vi "MAINrx.vi"() -> ()   [LabVIEW 2017]
uses:
  <instrlib>/niUSRP/niUSRP Write Tx Data (CDB).vi
panel:
  in  "SYNCHRO":i8[](array[numeric])=[0, 1, 1, 0, 1, 0, 0, 0, 0, 0, 0, 0, 1, 0, 0, 0, 0, 0, 1, 1]
  in  "simbol per write":i32=120
  out "Numeric":i32=3141
  out "cicli 2":dbl=18.0
  out "cicli":dbl=19.0
  in  "Silent symbol":i32=70
  in  "trama length":i32=20000
  out "original data  array":u16[](array[numeric])
  out "size(s)":i32=375000
  in  "Color":bool=TRUE
  out "Image out":T1(plugin-control)
  in  "Enabled Channel":string(combo)="0"
  in  "Device Name":refnum<k15>="192.168.10.2"
  in  "Active Antenna":string="TX1"
  in  "Gain":dbl=100.0 format="%#_6f"
  in  "Carrier Frequency":dbl format="%#_6p"
  in  "IQ Rate":dbl=2000000.0 format="%#_6p"
  in  "File Path":path=path "C:/Users/33769/Desktop/San-Giovanni-in-Fiore-Cosenza.jpg"
  in  "M":i32=16
  in  "pulse duration":i32=5
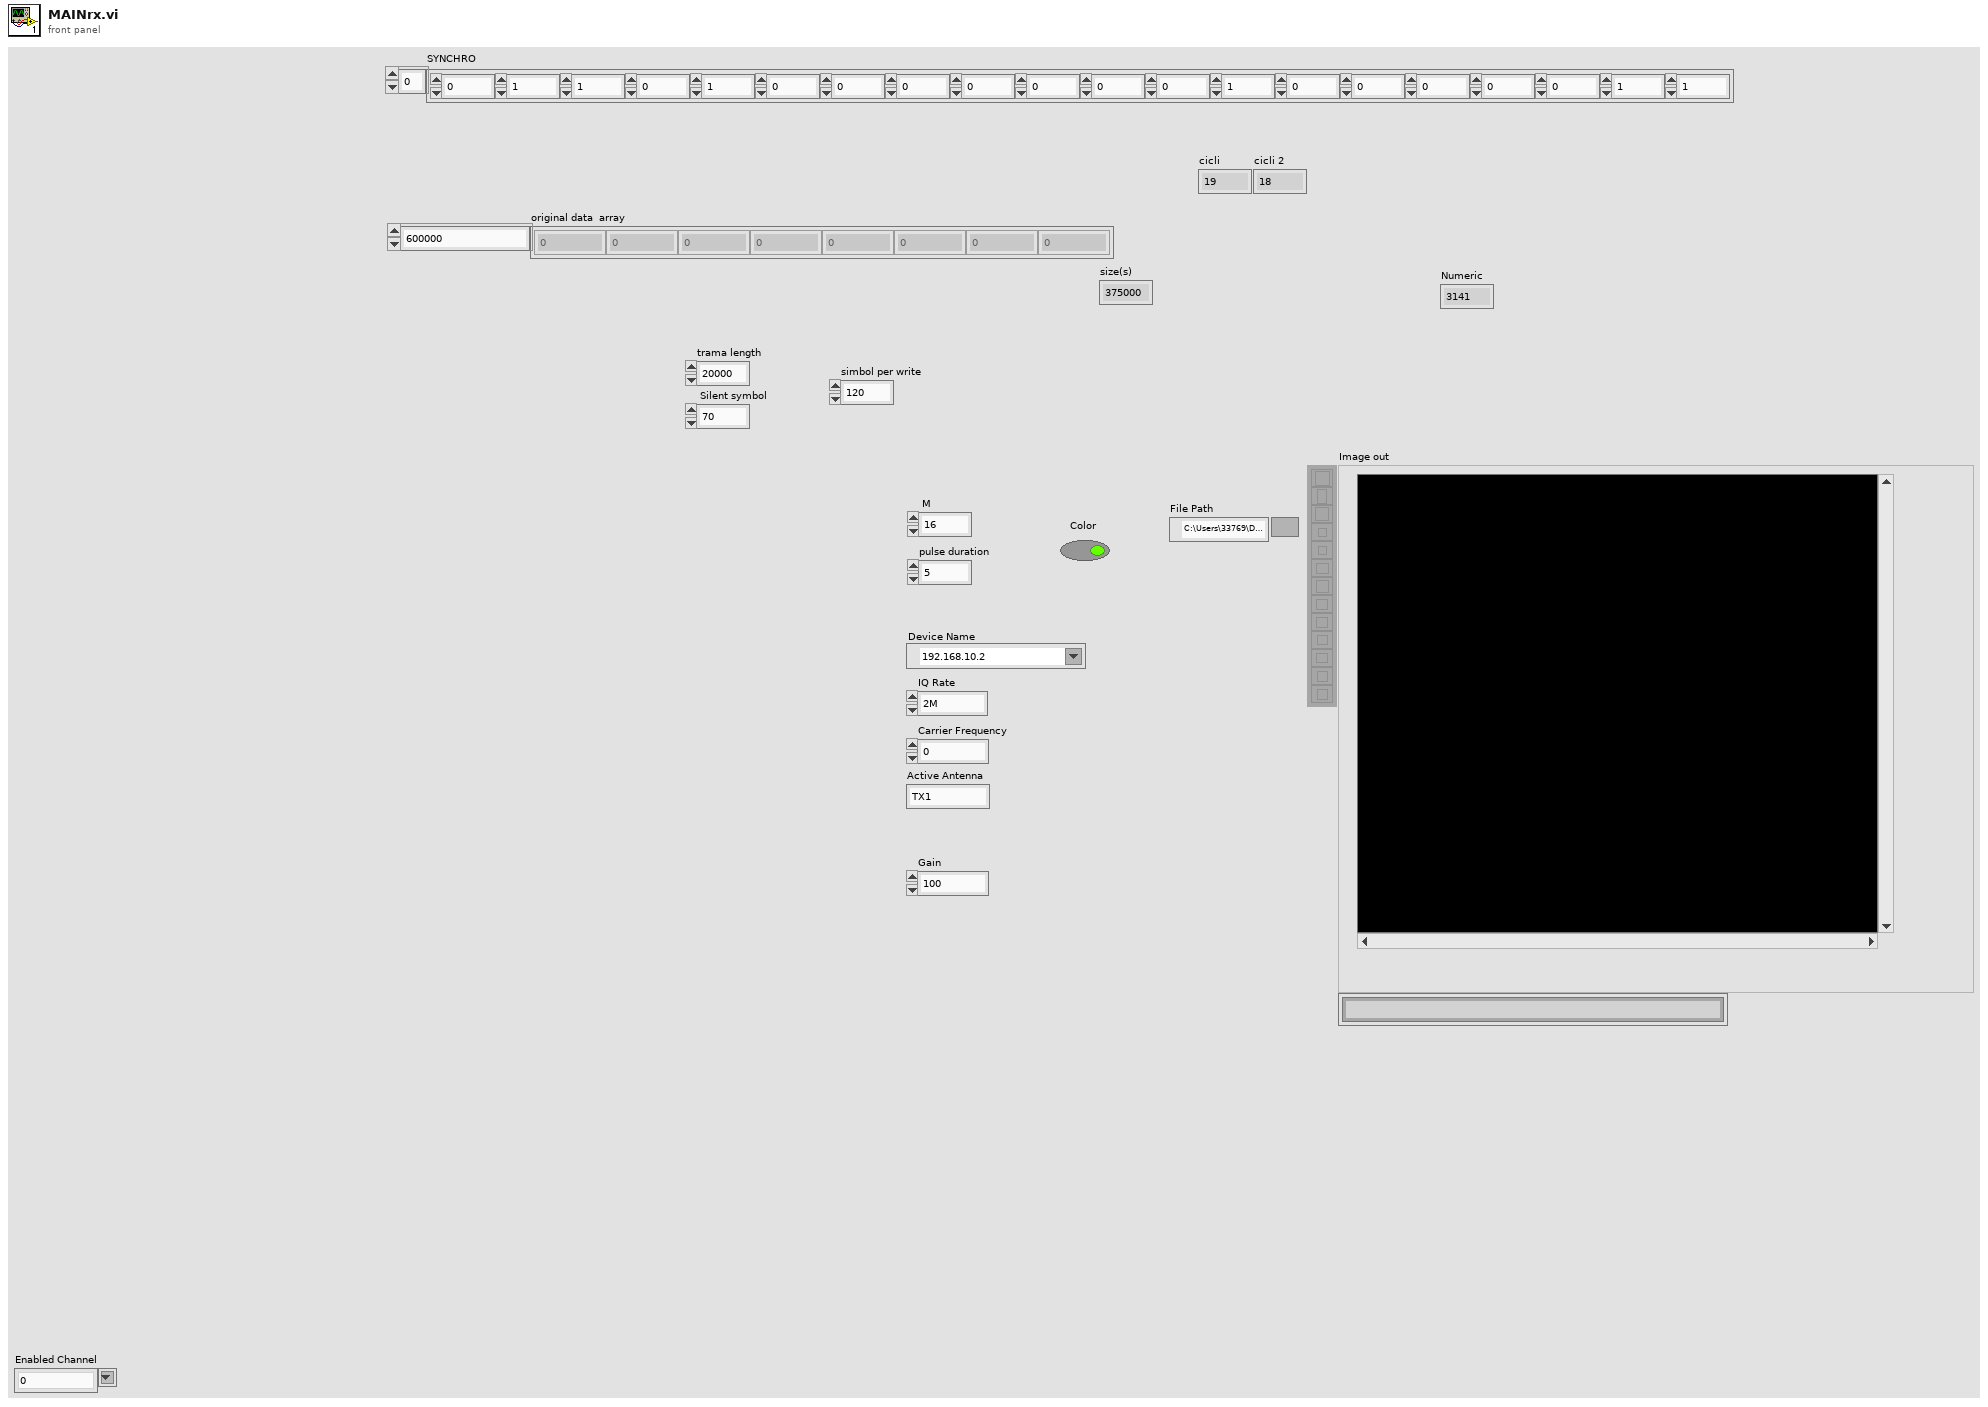
[diagram p1: front panel]
types:
  T1 = typedef "IMAQ Image.ctl" = refnum<image>
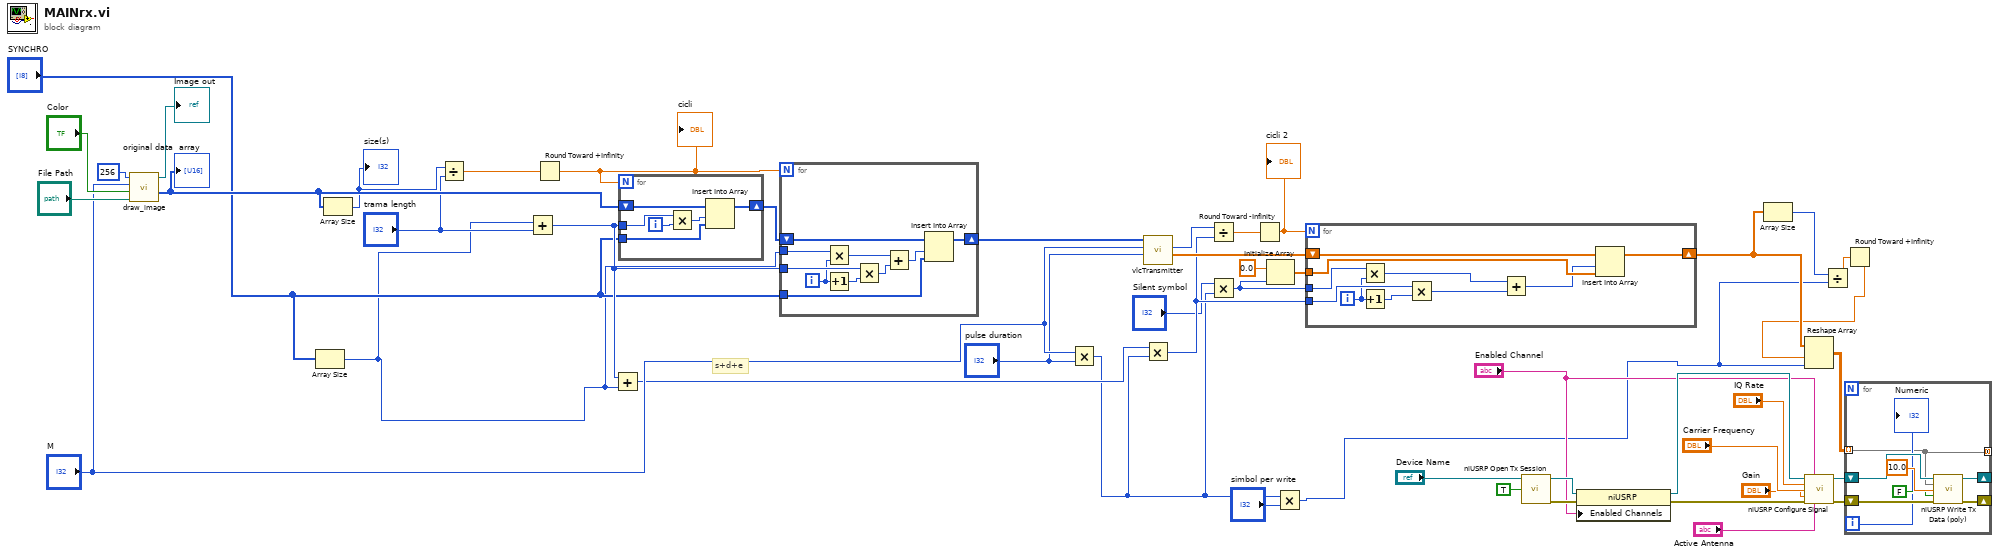
[diagram p0: block diagram]
diagram:
  # "s+d+e"
  n1 = call "draw_image.vi"("File Path"="File Path", "Color"="Color", "M"="M", "max"=i16 256) -> ("Array"=w29:u16[], "Image out"=→"Image out":T1)  [unwired: 6 in]
  "original data  array" <- w29
  n2 = Array Size(array="SYNCHRO") -> (size(s)=w1:i32)
  n3 = Array Size(array=w29) -> (size(s)=w15:i32)
  "size(s)" <- w15
  n4 = Divide(x=w15, y="trama length") -> (x/y=w16:dbl)
  n5 = Add(x=w1, y="trama length") -> (x+y=w13:i32)
  n6 = Round Toward +Infinity(x=w16) -> (ceil(x): smallest int >= x=w11:dbl)
  "cicli" <- w11
  n7 = Add(x=w13, y=w1) -> (x+y=w18:i32)
  n8 = for {
    N: w11 -> [_]
    tunnel: "SYNCHRO" -> [w53]
    shift-right: [w51] -> w12
    shift-left: w29 -> [w52]
    tunnel: w13 -> [w48]
    i -> [w50]
    n9 = Multiply(x=w48, y=w50) -> (x*y=w49:i32)
    n10 = Insert Into Array(array=w52, index=w49, new element=w53) -> (w51:u16[])
  }
  n11 = for {
    N: w11 -> [_]
    tunnel: "SYNCHRO" -> [w62]
    tunnel: w13 -> [w59]
    shift-right: [w63] -> w30
    shift-left: w12 -> [w61]
    tunnel: w1 -> [w55]
    i -> [w56]
    n12 = Multiply(x=w55, y=w56) -> (x*y=w57:i32)
    n13 = Increment(x=w56) -> (x+1=w60:i32)
    n14 = Multiply(x=w59, y=w60) -> (x*y=w58:i32)
    n15 = Add(x=w57, y=w58) -> (x+y=w54:i32)
    n16 = Insert Into Array(array=w61, index=w54, new element=w62) -> (w63:u16[])
  }
  n17 = Multiply(x="M", y="pulse duration") -> (x*y=w10:i32)
  n18 = call "vlcTransmitter.vi"("pulse duration"="pulse duration", "M"="M", "Array in"=w30) -> ("Array out"=w24:cdb[], "size(s)"=w23:i32)  [unwired: 7 in]
  n19 = Multiply(x=w18, y=w10) -> (x*y=w22:i32)
  n20 = Divide(x=w23, y=w22) -> (x/y=w21:dbl)
  n21 = Multiply(x="Silent symbol", y=w10) -> (x*y=w19:i32)
  n22 = Round Toward -Infinity(1:w21) -> (0:w20:dbl)
  "cicli 2" <- w20
  n23 = Initialize Array(0.0 ("element"), w19) -> (w27:dbl[])
  n24 = Multiply(x=w10, y="simbol per write") -> (x*y=w5:i32)
  n25 = for {
    N: w20 -> [_]
    tunnel: w27 -> [w73]
    tunnel: w22 -> [w69]
    shift-right: [w72] -> w7
    shift-left: w24 -> [w71]
    tunnel: w19 -> [w68]
    i -> [w67]
    n26 = Multiply(x=w68, y=w67) -> (x*y=w65:i32)
    n27 = Increment(x=w67) -> (x+1=w70:i32)
    n28 = Multiply(x=w69, y=w70) -> (x*y=w66:i32)
    n29 = Add(x=w65, y=w66) -> (x+y=w64:i32)
    n30 = Insert Into Array(array=w71, index=w64, new element=w73) -> (w72:cdb[])
  }
  n31 = call <instrlib>:"niUSRP Open Tx Session.vi"("device names"="Device Name", "reset"=TRUE) -> ("session handle out"=w39:refnum<k15>, "error out"=w40:errorcluster)  [unwired: 12 in]
  n32 = property class="niUSRP"(reference=w39, error in=w40, "Enabled Channels"="Enabled Channel") -> (reference out=w38:refnum<k15>, error out=w37:errorcluster)
  n33 = Array Size(array=w7) -> (size(s)=w6:i32)
  n34 = call <instrlib>:"niUSRP Configure Signal.vi"("session handle"=w38, "channel list"="Enabled Channel", "IQ rate"="IQ Rate", "carrier frequency"="Carrier Frequency", "gain"="Gain", "error in (no error)"=w37, "active antenna"="Active Antenna") -> ("session handle out"=w33:refnum<k15>, "error out"=w34:errorcluster)  [unwired: 4 in, 3 out]
  n35 = Divide(x=w6, y=w5) -> (x/y=w4:dbl)
  n36 = Round Toward +Infinity(x=w4) -> (ceil(x): smallest int >= x=w3:dbl)
  n37 = Reshape Array(w7, w3, w5) -> (w8:cdb[][])
  n38 = for {
    tunnel: w8 -> [w74] mode=indexing
    shift-right: [w80] -> _
    shift-left: w34 -> [w77]
    shift-right: [w81] -> _
    shift-left: w33 -> [w76]
    tunnel: [w74] -> _ mode=concatenating
    i -> [w75]
    n39 = call-poly <instrlib>:"niUSRP Write Tx Data (poly).vi"("session handle"=w76, "data"=w74, "timeout"=10.0, "end of data?"=FALSE, "error in (no error)"=w77) -> ("session handle out"=w81:refnum<k15>, "error out"=w80:errorcluster)  [unwired: 9 in]
    "Numeric" <- w75
  }
